vi "Close.vi"(8 "error in (no error)":errorcluster, 11 "Keysight44xx in":refnum<class "Keysight44xx.lvclass">) -> (0 "error out":errorcluster, 3 "Keysight44xx out":refnum<class "Keysight44xx.lvclass">)   [LabVIEW 2018, in "SpecAnPlugins.lvlib" / "Keysight44xx.lvclass"]
doc: "This function closes the reference to the instrument and sets the connected boolean to false."
uses:
  Keysight44xx.lvclass
  C:/Users/ico/Documents/Projects/NistPluggableModules/SpecAn/SpecAnPlugins/SpecAnBaseClass/SpecAnBase.lvclass
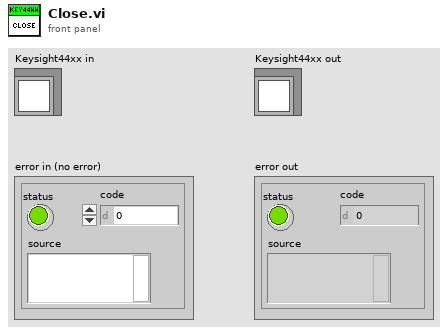
[diagram p1: front panel]
types:
  T1 = typedef "SpecAnPlugins.lvlib/SpecAnBase.lvclass/Acquisition.ctl" = cluster{"Handle":string, "Connected":bool, "Enabled":bool, "SweepModeContinuous":bool, "NumberOfSweeps":i32, "DetectorTypeAuto":bool, "DetectorType":i32, "VerticalScale":i32, "MaximumTime(seconds)":dbl}
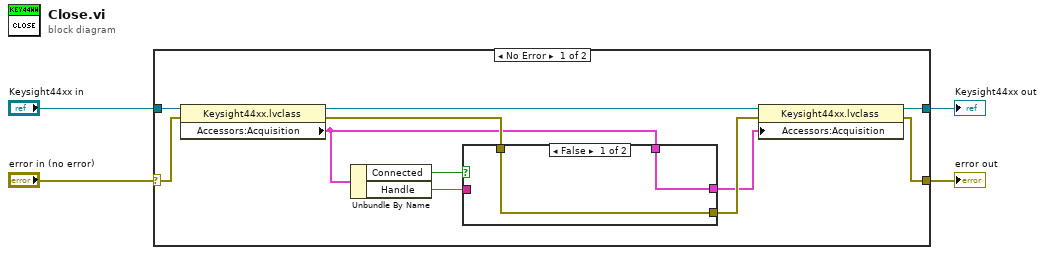
[diagram p0: block diagram]
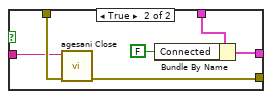
[diagram p2: hidden frame]
diagram:
  n1 = case shown="No Error" "error in (no error)" {
    selector: "error in (no error)" -> [w14 w24]
    tunnel: "Keysight44xx in" -> [w15 w25]
    tunnel: [w10 w25] -> w2
    tunnel: [w9 w24] -> w1
    frame No Error {
      n2 = property class="Keysight44xx.lvclass"(reference=w15, error in=w14) -> (reference out=w11:refnum<class "Keysight44xx.lvclass">, error out=w13:errorcluster, "Accessors:Acquisition"=w7:T1)
      n3 = Unbundle By Name(w7) -> ("Connected"=w5:bool, "Handle"=w12:string)
      n4 = case shown="False" w5 {
        tunnel: w13 -> [w16 w23]
        tunnel: w12 -> [_ w22]
        tunnel: [w16 w21] -> w8
        tunnel: w7 -> [w17 w20]
        tunnel: [w17 w19] -> w6
        frame False {
        }
        frame True {
          n5 = call <instrlib>:"agesani Close.vi"("error in (no error)"=w23, "instrument handle"=w22) -> ("error out"=w21:errorcluster)  [unwired: 9 out]
          n6 = Bundle By Name(cluster=w20, "Connected"=FALSE) -> (w19:T1)
        }
      }
      n7 = property class="Keysight44xx.lvclass"(reference=w11, error in=w8, "Accessors:Acquisition"=w6) -> (reference out=w10:refnum<class "Keysight44xx.lvclass">, error out=w9:errorcluster)
    }
    frame Error {
    }
  }
  "error out" <- w1
  "Keysight44xx out" <- w2
